vi "dfd_Convert INT SOS Coefficients to String.vi"(5 "indent order":i32, 6 "width (a)":i16, 7 "width (b)":i16, 9 "1":i32, 10 "coef a":i32[](array[numeric]), 11 "coef b":i32[](array[numeric])) -> (3 "XML string out":string)   [LabVIEW 2017, in "NI_DigFilter_Process.lvlib"]
uses:
  <vilib>/addons/Digital Filter Design/NI_DigFilter_Process.lvlib
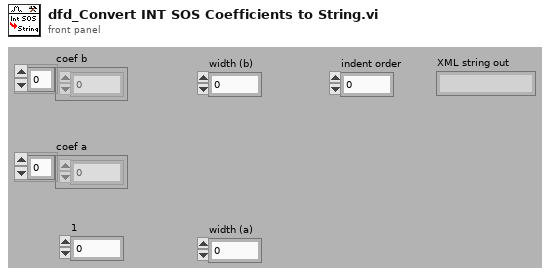
[diagram p1: front panel]
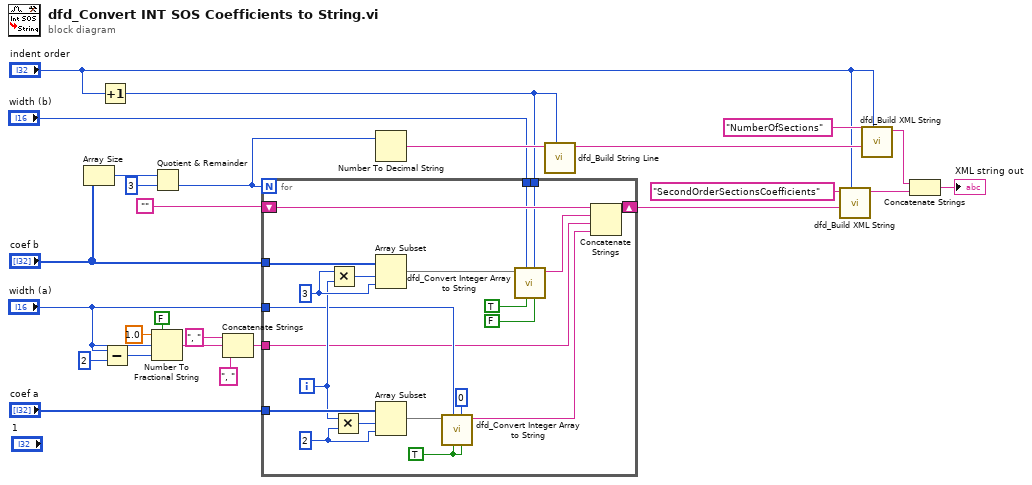
[diagram p0: block diagram]
diagram:
  n1 = Array Size(array="coef b") -> (size(s)=w26:i32)
  n2 = Increment(x="indent order") -> (x+1=w4:i32)
  n3 = Subtract(x="width (a)", y=i16 2) -> (x-y=w8:i16)
  n4 = Number To Fractional String(use system decimal point (T)=FALSE, number=1.0, width (-)="width (a)", precision (6)=w8) -> (F-format string=w5:string)
  n5 = Quotient & Remainder(x=w26, y=3) -> (floor(x/y)=w17:i32)  [unwired: 1 out]
  n6 = Concatenate Strings(", " ("string"), w5, ", " ("string")) -> (w3:string)
  n7 = for {
    N: w17 -> [_]
    tunnel: "coef a" -> [w47]
    tunnel: "coef b" -> [w44]
    shift-right: [w37] -> w21
    shift-left: "" -> [w42]
    tunnel: w4 -> [w32]
    tunnel: "width (b)" -> [w35]
    tunnel: "width (a)" -> [w36]
    tunnel: w3 -> [w28]
    i -> [w40]
    w29 = TRUE
    w43 = 3 ("y")
    w41 = 2 ("y")
    n8 = Multiply(x=w43, y=w40) -> (x*y=w45:i32)
    n9 = Multiply(x=w40, y=w41) -> (x*y=w46:i32)
    n10 = Array Subset(array=w44, index=w45, length=w43) -> (w39:i32[])
    n11 = Array Subset(array=w47, index=w46, length=w41) -> (w34:i32[])
    n12 = call <vilib>:"dfd_Convert Integer Array to String.vi"("append EOL?"=w29, "indent order"=0, "display in one line?"=w29, "width (-)"=w36, "I32 values"=w34) -> ("string"=w27:string)  [unwired: 6 out]
    n13 = call <vilib>:"dfd_Convert Integer Array to String.vi"("append EOL?"=FALSE, "indent order"=w32, "display in one line?"=TRUE, "width (-)"=w35, "I32 values"=w39) -> ("string"=w38:string)  [unwired: 6 out]
    n14 = Concatenate Strings(w42, w38, w28, w27) -> (w37:string)
  }
  n15 = Number To Decimal String(number=w17) -> (decimal integer string=w18:string)  [unwired: 1 out]
  n16 = call <vilib>:"dfd_Build String Line.vi"("indent order"=w4, "string"=w18) -> ("string line"=w19:string)  [unwired: 9 out]
  n17 = call <vilib>:"dfd_Build XML String.vi"("indent order"="indent order", "string in"=w21, "element name"="SecondOrderSectionsCoefficients") -> ("xml string out"=w23:string)  [unwired: 1 in, 7 out]
  n18 = call <vilib>:"dfd_Build XML String.vi"("indent order"="indent order", "string in"=w19, "element name"="NumberOfSections") -> ("xml string out"=w20:string)  [unwired: 1 in, 7 out]
  n19 = Concatenate Strings(w20, w23) -> (→"XML string out":string)
